vi "LVUT_MainSequence(Simple Example_Station2).vi"(8 "error in (no error)":errorcluster) -> (0 "error out":errorcluster)   [LabVIEW 2019, in "Simple Example(Station2).lvlib"]
uses:
  Simple Example(Station2).lvlib
  Unit Test Engine Tools.lvlib
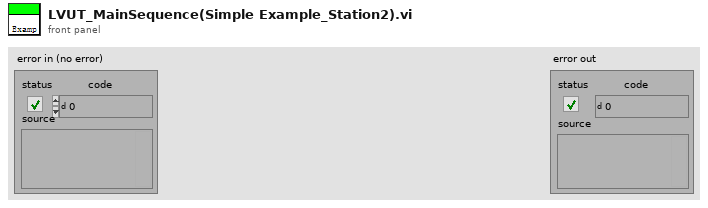
[diagram p1: front panel]
types:
  T1 = enum16{"Station 1", "Station 2", "Station 3", "Station 4"}
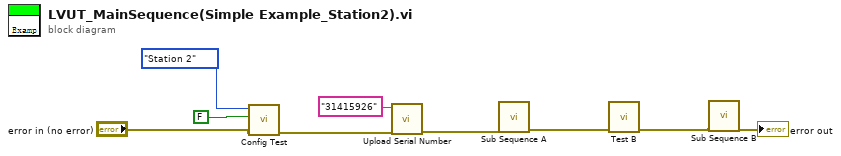
[diagram p0: block diagram]
diagram:
  n1 = call "Config Test.vi"("Error In"="error in (no error)", "Debug"=FALSE, "Station"=T1."Station 2") -> ("Error Out"=w2:errorcluster)  [unwired: 8 in]
  n2 = call "Upload Serial Number.vi"("error in (no error)"=w2, "SerialNumber"="31415926") -> ("error out"=w1:errorcluster)  [unwired: 9 in]
  n3 = call "Sub Sequence A.vi"("error in (no error)"=w1) -> ("error out"=w7:errorcluster)  [unwired: 10 in]
  n4 = call "Test B.vi"("error in (no error)"=w7) -> ("error out"=w8:errorcluster)  [unwired: 10 in]
  n5 = call "Sub Sequence B.vi"("error in (no error)"=w8) -> ("error out"=→"error out":errorcluster)  [unwired: 10 in]
